vi "random_access_write.vi"(10 "address in":u32) -> (2 "address out":u32, 4 "FIFO scan time out":bool)   [LabVIEW 2010]
uses:
  <vilib>/rvi/DataTransferAndStorage/Container/XNode/niFpgaContainer.xnode
  <vilib>/rvi/DataTransferAndStorage/Container/Common/niFpgaContainerMethod.ctl
  <vilib>/rvi/DataTransferAndStorage/Container/Common/niFpgaTransferTypeControl.ctl
  <vilib>/rvi/interface/RandomDataEmulation/nirviRandomDataFPGAFIFO.vi
  <vilib>/rvi/interface/RandomDataEmulation/niFpgaRandomDataHandleErrors.vi
  <vilib>/rvi/Memory/Memory_Emulation/nirvimemoryEmulationManagerCache_GetValue.vi
  <vilib>/rvi/DataTransferAndStorage/Container/Common/niFpgaContainerGetUniqueNameForEmu.vi
  <vilib>/rvi/Memory/Memory_Emulation/nirvimemoryEmulationManagerCache_InsertValue.vi
  <vilib>/Utility/error.llb/Clear Errors.vi
  <vilib>/rvi/Memory/Memory_Emulation/nirvimemoryEmulationManagerCache_SetValue.vi
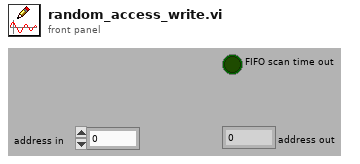
[diagram p1: front panel]
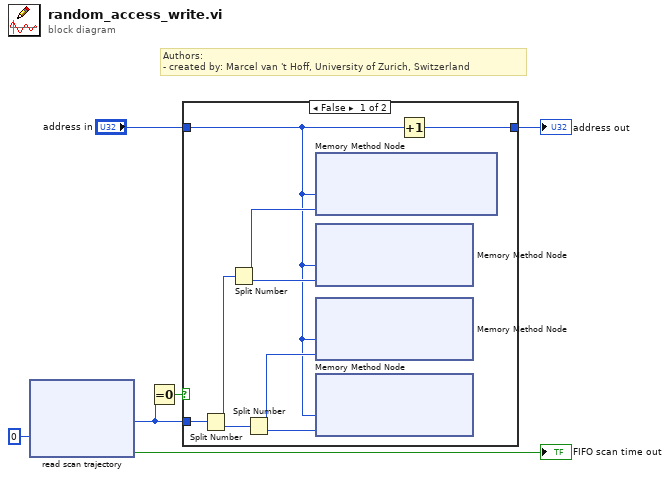
[diagram p0: block diagram]
diagram:
  # "Authors: \n- created by: Marcel van 't Hoff, University of Zurich, Switzerland"
  n1 = xnode "read scan trajectory"("Timeout"=0) -> ("Element"=w2:u64, "Timed Out?"=→"FIFO scan time out":bool)  [unwired: 1 in, 1 out]
  n2 = Equal To 0?(x=w2) -> (x = 0?=w4:bool)
  n3 = case shown="False" w4 {
    tunnel: w2 -> [w15 _]
    tunnel: "address in" -> [w7 w516]
    tunnel: [w11 w516] -> w6
    frame False {
      n4 = Split Number(x=w15) -> (hi(x)=w14:u32, lo(x)=w10:u32)
      n5 = Split Number(x=w14) -> (hi(x)=w13:u16, lo(x)=w12:u16)
      n6 = Split Number(x=w10) -> (hi(x)=w9:u16, lo(x)=w8:u16)
      n7 = xnode ("Memory Method Node")("Address"=w7, "Data"=w13) -> ()  [unwired: 1 in, 1 out]
      n8 = xnode ("Memory Method Node")("Address"=w7, "Data"=w12) -> ()  [unwired: 1 in, 1 out]
      n9 = xnode ("Memory Method Node")("Address"=w7, "Data"=w9) -> ()  [unwired: 1 in, 1 out]
      n10 = xnode ("Memory Method Node")("Address"=w7, "Data"=w8) -> ()  [unwired: 1 in, 1 out]
      n11 = Increment(x=w7) -> (x+1=w11:u32)
    }
    frame True {
    }
  }
  "address out" <- w6
